vi "OpenInterface.vi"(10 "nIndex":u32, 11 "error in (no error)":errorcluster) -> (1 "return type":i32, 2 "hIFDev":i64, 3 "error out":errorcluster)   [LabVIEW 2016]
uses:
  MVSDKmd.dll
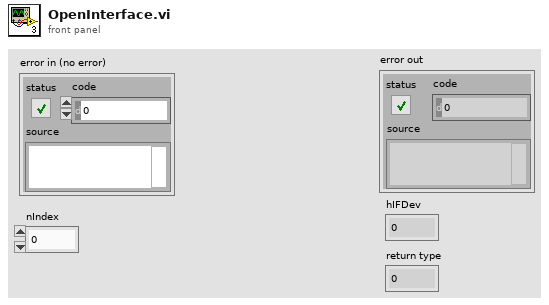
[diagram p1: front panel]
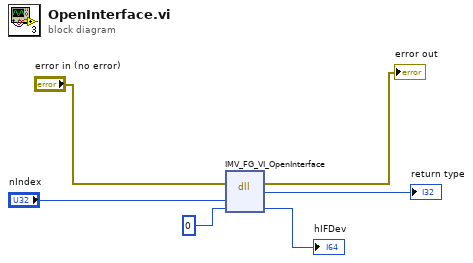
[diagram p0: block diagram]
diagram:
  n1 = dll-call lib="MVSDKmd.dll" fn="IMV_FG_VI_OpenInterface"(error in="error in (no error)", "nIndex"="nIndex", "hIFDev"=i64 0) -> (error out=→"error out":errorcluster, "return type"=→"return type":i32, "hIFDev"=→"hIFDev":i64)  [unwired: 3 in, 1 out]
